vi "DifferentStdPrototype.vi"(3 "Input buffer":T3, 4 "Sequence Context":T1) -> (0 "error out":errorcluster, 1 "Test Data":T2 {"Numeric Measurement" format="%.2f"})   [LabVIEW 2009]
uses:
  LabVIEW Test - Input Buffer.ctl
  LabVIEW Test - Test Data.ctl
  LabVIEW Test - Sequence Context.ctl
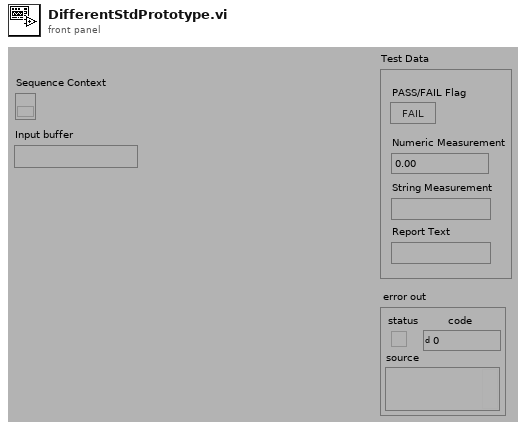
[diagram p1: front panel]
types:
  T1 = typedef "LabVIEW Test - Sequence Context.ctl" = refnum<k7>
  T2 = typedef "LabVIEW Test - Test Data.ctl" = cluster{"PASS/FAIL Flag":bool, "Numeric Measurement":dbl, "String Measurement":string, "Report Text":string}
  T3 = typedef "LabVIEW Test - Input Buffer.ctl" = string
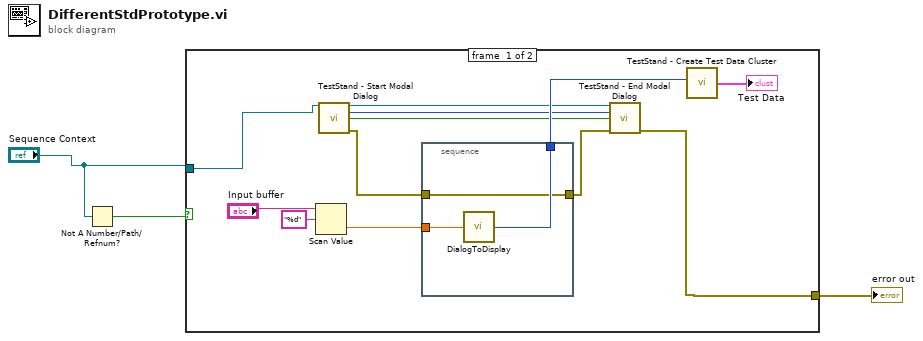
[diagram p0: block diagram]
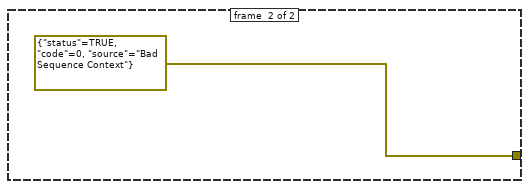
[diagram p2: hidden frame]
diagram:
  n1 = Not A Number/Path/Refnum?(number/path/refnum="Sequence Context") -> (NaN/Path/Refnum?=w2:bool)
  n2 = case shown="False" w2 {
    tunnel: "Sequence Context" -> [w5 _]
    tunnel: [w4 errorcluster {"status"=TRUE, "code"=0, "source"="Bad Sequence Context"} ("error out")] -> w1
    frame #0 {
      n3 = Scan Value(string="Input buffer", format string="%d") -> (value=w12:dbl)  [unwired: 1 in, 1 out]
      n4 = call "TestStand - Start Modal Dialog.vi"("Sequence Context In"=w5) -> ("Sequence Context Out"=w10:T1, "Modal ID"=w8:i32, "VI Originally Open"=w7:bool, "error out"=w6:errorcluster)  [unwired: 10 in, 1 out]
      n5 = stacked-sequence {
        tunnel: w12 -> [w18]
        tunnel: [w17] -> w11
        tunnel: w6 -> [w16]
        tunnel: [w16] -> w9
        frame #0 {
          n6 = call "DialogToDisplay.vi"("Numeric"=w18) -> ("Numeric 2"=w17:i32)
        }
      }
      n7 = call "TestStand - End Modal Dialog.vi"("Sequence Context In"=w10, "Modal ID"=w8, "VI Originally Open"=w7, "error in (no error)"=w9) -> ("error out"=w4:errorcluster)  [unwired: 11 in]
      n8 = call "TestStand - Create Test Data Cluster.vi"("Numeric Measurement"=w11) -> ("Test Data"=→"Test Data":T2)  [unwired: 3 in]
    }
    frame #1 {
    }
  }
  "error out" <- w1
